vi "TSL_Information.vi"(0 ".NET Reference in":refnum<k24>, 7 "error in (no error)":errorcluster) -> (9 "ProductName":string, 11 "SerialNumber":string, 12 "MaximumSpeed":dbl, 13 "FWversion":string, 14 "MinimumSpeed":dbl, 16 "MinimunWavelength":dbl, 17 "MinimumATTValue":dbl, 18 "MaximumWavelength":dbl, 19 "MaximumATTValue":dbl, 20 "Reference out":refnum<k24>, 21 "MaximumFrequency":dbl, 22 "MinimunFrequency":dbl, 23 "MinimumAPCPower_dBm":dbl, 24 "MaximumAPCPower_dBm":dbl, 25 "MinimumAPCPower_mW":dbl, 26 "MaximumAPCPower_mW":dbl, 27 "error out":errorcluster)   [LabVIEW 2017]
uses:
  C:/Users/Ssantec_Test/Documents/Instrument_DLL_Sample_Labview_20220902_Ver1.2.2/DLL/x86/InstrumentDLL.dll
  DLL/x86/InstrumentDLL.dll
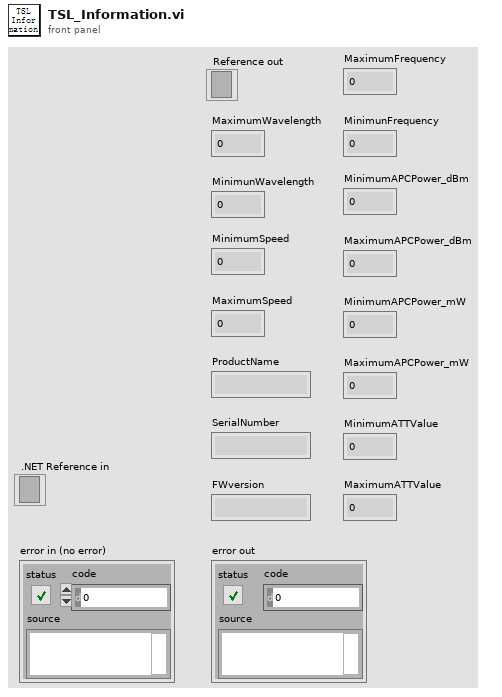
[diagram p1: front panel]
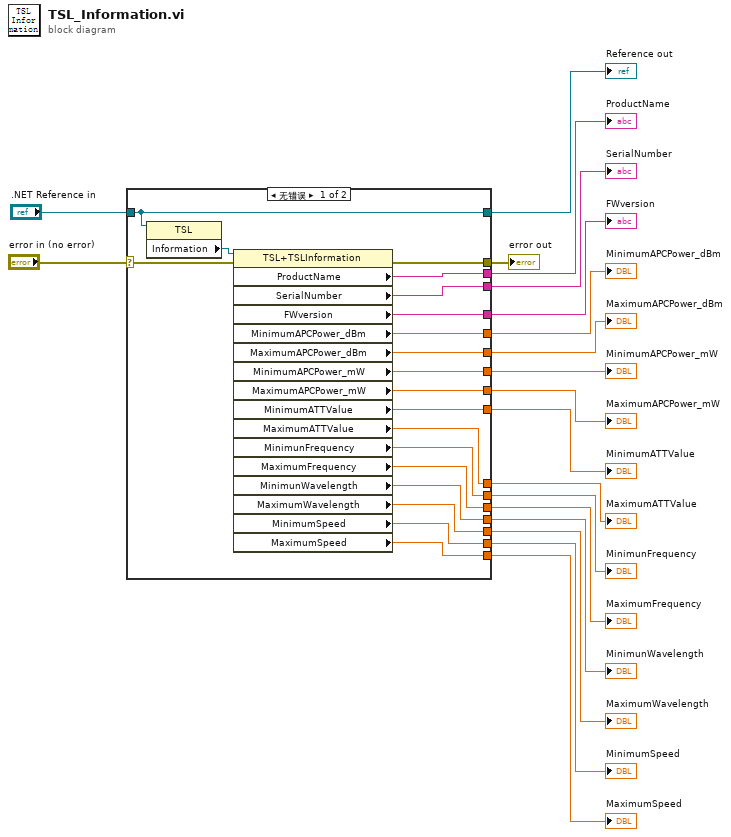
[diagram p0: block diagram]
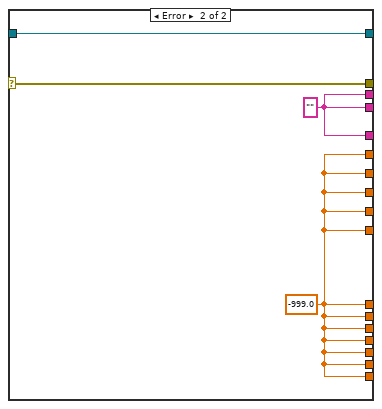
[diagram p2: hidden frame]
diagram:
  n1 = case shown="无错误" "error in (no error)" {
    selector: "error in (no error)" -> [w22 w42]
    tunnel: [w38 w41] -> w19
    tunnel: [w37 w41] -> w18
    tunnel: [w36 w41] -> w17
    tunnel: [w35 w41] -> w16
    tunnel: [w34 w41] -> w15
    tunnel: [w33 w41] -> w14
    tunnel: [w32 w41] -> w13
    tunnel: [w31 w41] -> w12
    tunnel: [w30 w41] -> w11
    tunnel: [w29 w41] -> w10
    tunnel: [w28 w41] -> w9
    tunnel: [w27 w41] -> w8
    tunnel: ".NET Reference in" -> [w20 w40]
    tunnel: [w26 w39] -> w7
    tunnel: [w25 w39] -> w6
    tunnel: [w24 w39] -> w5
    tunnel: [w23 w42] -> w4
    tunnel: [w20 w40] -> w1
    frame No Error {
      n2 = property on="属性节点" class="TSL"(reference=w20) -> ("Information"=w21:refnum<k24>)  [unwired: 1 in, 2 out]
      n3 = property on="属性节点" class="TSL+TSLInformation"(reference=w21, error in=w22) -> (error out=w23:errorcluster, "ProductName"=w26:string, "SerialNumber"=w25:string, "FWversion"=w24:string, "MinimumAPCPower_dBm"=w30:dbl, "MaximumAPCPower_dBm"=w29:dbl, "MinimumAPCPower_mW"=w28:dbl, "MaximumAPCPower_mW"=w27:dbl, "MinimumATTValue"=w32:dbl, "MaximumATTValue"=w31:dbl, "MinimunFrequency"=w34:dbl, "MaximumFrequency"=w33:dbl, "MinimunWavelength"=w36:dbl, "MaximumWavelength"=w35:dbl, "MinimumSpeed"=w37:dbl, "MaximumSpeed"=w38:dbl)  [unwired: 1 out]
    }
    frame Error {
      w41 = -999.0 ("MinimumAPCPower_dBm")
      w39 = "" ("ProductName")
    }
  }
  "MaximumSpeed" <- w19
  "MinimumSpeed" <- w18
  "MinimunWavelength" <- w17
  "MaximumWavelength" <- w16
  "MinimunFrequency" <- w15
  "MaximumFrequency" <- w14
  "MinimumATTValue" <- w13
  "MaximumATTValue" <- w12
  "MinimumAPCPower_dBm" <- w11
  "MaximumAPCPower_dBm" <- w10
  "MinimumAPCPower_mW" <- w9
  "MaximumAPCPower_mW" <- w8
  "ProductName" <- w7
  "SerialNumber" <- w6
  "FWversion" <- w5
  "error out" <- w4
  "Reference out" <- w1
